vi "Append_Array_2D.vi"(1 "Array to append":dbl[][](array[numeric]), 2 "Array in":dbl[][](array[numeric])) -> (0 "Array out":dbl[][](array[numeric]))   [LabVIEW 2015]
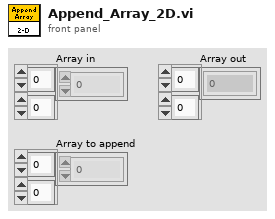
[diagram p1: front panel]
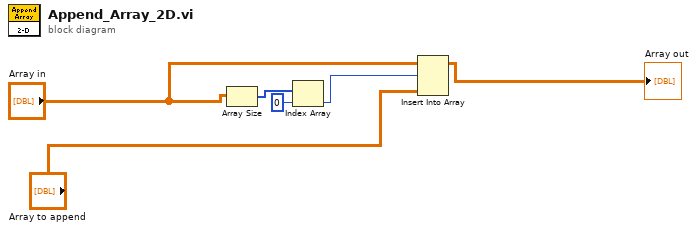
[diagram p0: block diagram]
diagram:
  n1 = Array Size(array="Array in") -> (size(s)=w3:i32[])
  n2 = Index Array(array=w3, index=0) -> (element=w5:i32)
  n3 = Insert Into Array(array="Array in", index (row)=w5, new element="Array to append") -> (→"Array out":dbl[][])  [unwired: 1 in]
